vi "Do Action.vi"(4 "error in (no error)":errorcluster, 6 "Array in":refnum<class>[](array[class]), 7 "Act_Increment All in":refnum<class "Act_Increment All.lvclass">) -> (0 "error out":errorcluster, 2 "Array out":refnum<class>[](array[class]), 3 "Act_Increment All out":refnum<class "Act_Increment All.lvclass">)   [LabVIEW 2014, in "Act_Increment All.lvclass"]
uses:
  Act_Increment All.lvclass
  Data/Data.lvclass
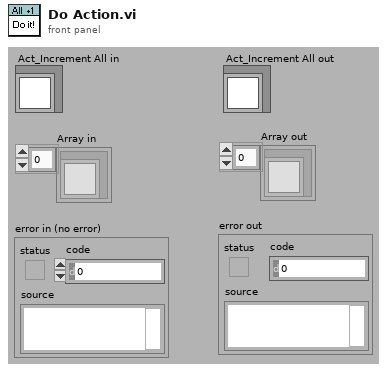
[diagram p1: front panel]
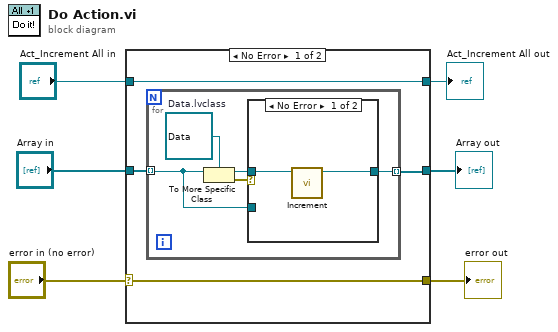
[diagram p0: block diagram]
diagram:
  n1 = case shown="No Error" "error in (no error)" {
    selector: "error in (no error)" -> [w8 w20]
    tunnel: "Array in" -> [w9 w19]
    tunnel: "Act_Increment All in" -> [w10 w21]
    tunnel: [w10 w21] -> w3
    tunnel: [w8 w20] -> w2
    tunnel: [w7 w19] -> w1
    frame No Error {
      n2 = for {
        tunnel: w9 -> [w11] mode=indexing
        tunnel: [w12] -> w7 mode=indexing
        w15 = refnum<class "Data.lvclass"> refnum  # Data.lvclass
        n3 = To More Specific Class(target class=w15, reference=w11) -> (specific class reference=w13:refnum<class "Data.lvclass">, error out=w14:errorcluster)  [unwired: 1 in]
        n4 = case shown="No Error" w14 {
          tunnel: w13 -> [w17 _]
          tunnel: [w16 w18] -> w12
          tunnel: w11 -> [_ w18]
          frame No Error {
            n5 = call-dynamic "Increment.vi"("Data in"=w17) -> ("Data out"=w16:refnum<class "Data.lvclass">)  [unwired: 9 in, 1 out]
          }
          frame Error {
          }
        }
      }
    }
    frame Error {
    }
  }
  "error out" <- w2
  "Array out" <- w1
  "Act_Increment All out" <- w3
